vi "test.vi"() -> ()   [LabVIEW 2013]
panel:
  out "error out 2":errorcluster
  out "connection ID":refnum<k5>
  out "Numeric":i32
  out "error out":errorcluster
  in  "stop":bool
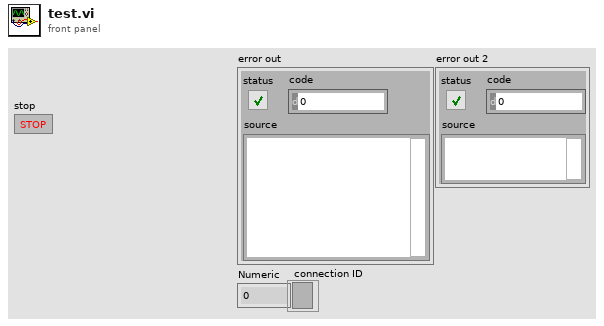
[diagram p1: front panel]
types:
  T1 = enum16{"Standard", "Buffered", "CRLF", "Immediate"}
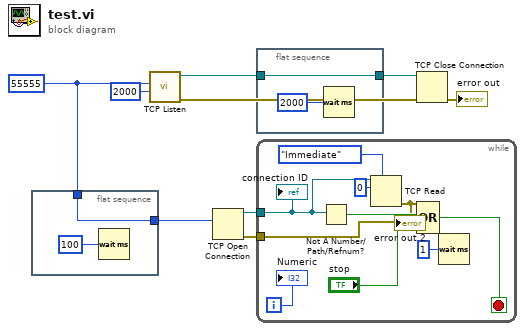
[diagram p0: block diagram]
diagram:
  w3 = u16 55555 ("remote port or service name")
  n1 = flat-sequence {
    tunnel: w3 -> [w10]
    tunnel: [w10] -> w8
    frame #0 {
      n2 = Wait (ms)(milliseconds to wait=u32 100) -> ()  [unwired: 1 out]
    }
  }
  n3 = call <vilib>:"TCP Listen.vi"("timeout ms (wait forever: -1)"=2000, "port"=w3) -> ("error out"=w2:errorcluster, "connection ID"=w4:refnum<k5>)  [unwired: 5 in, 3 out]
  n4 = TCP Open Connection(remote port or service name=w8) -> (connection ID=w9:refnum<k5>, error out=w5:errorcluster)  [unwired: 4 in]
  n5 = flat-sequence {
    tunnel: [w12] -> w7
    tunnel: w4 -> [w12]
    frame #0 {
      n6 = Wait (ms)(milliseconds to wait=u32 2000) -> ()  [unwired: 1 out]
    }
  }
  n7 = while {
    tunnel: w9 -> [w17]
    tunnel: w5 -> [w19]
    i -> [w18]
    stop <- w21 stop-if-true
    n8 = Not A Number/Path/Refnum?(number/path/refnum=w17) -> (NaN/Path/Refnum?=w23:bool)
    n9 = TCP Read(connection ID=w17, bytes to read=0, 7:T1."Immediate" ("mode (standard)")) -> (error out=w14:errorcluster)  [unwired: 2 in, 2 out]
    "error out 2" <- w14
    n10 = Compound Arithmetic op=OR(w14, w23, w19, "stop") -> (w21:bool)
    n11 = Wait (ms)(milliseconds to wait=u32 1) -> ()  [unwired: 1 out]
    "Numeric" <- w18
    "connection ID" <- w17
  }
  n12 = TCP Close Connection(connection ID=w7, error in (no error)=w2) -> (error out=→"error out":errorcluster)  [unwired: 1 in, 1 out]
